vi "Set Metadata.vi"(9 "Metadata Disable":T2={"spectrometer"=enum."Disabled and Grayed Out", "sphere"=enum."Disabled and Grayed Out", "analyzer"=enum."Disabled and Grayed Out", "ampGainRange"=enum."Disabled and Grayed Out"}, 11 "Data Fields":T1={"operatorName"="", "project"="", "measurementType"="", "sphere"="", "spectrometer"="", "powerSource"="", "analyzer"="", "fixtureType"="", "lampType"="", "sourceType"="", "testOrientation"="", "model"="", "sample"="", "hours"=".csv", "Amp Gain Range"=""}) -> (3 "Metadata Out":string[][](array[string]))   [LabVIEW 2013]
uses:
  Metadata disable typedef.ctl
  Metadata typedef.ctl
panel:
  in  "Ready?":bool
  out "data string":string
  # "ambient temp (sphere)"
  # "ambient temp room"
  # "Fill out the follow data fields for each test. An error will be thrown if any data fields are missing.\nNew parameters for data fields can be added by right clicking, hitting \"properties\", then \"edit items\""
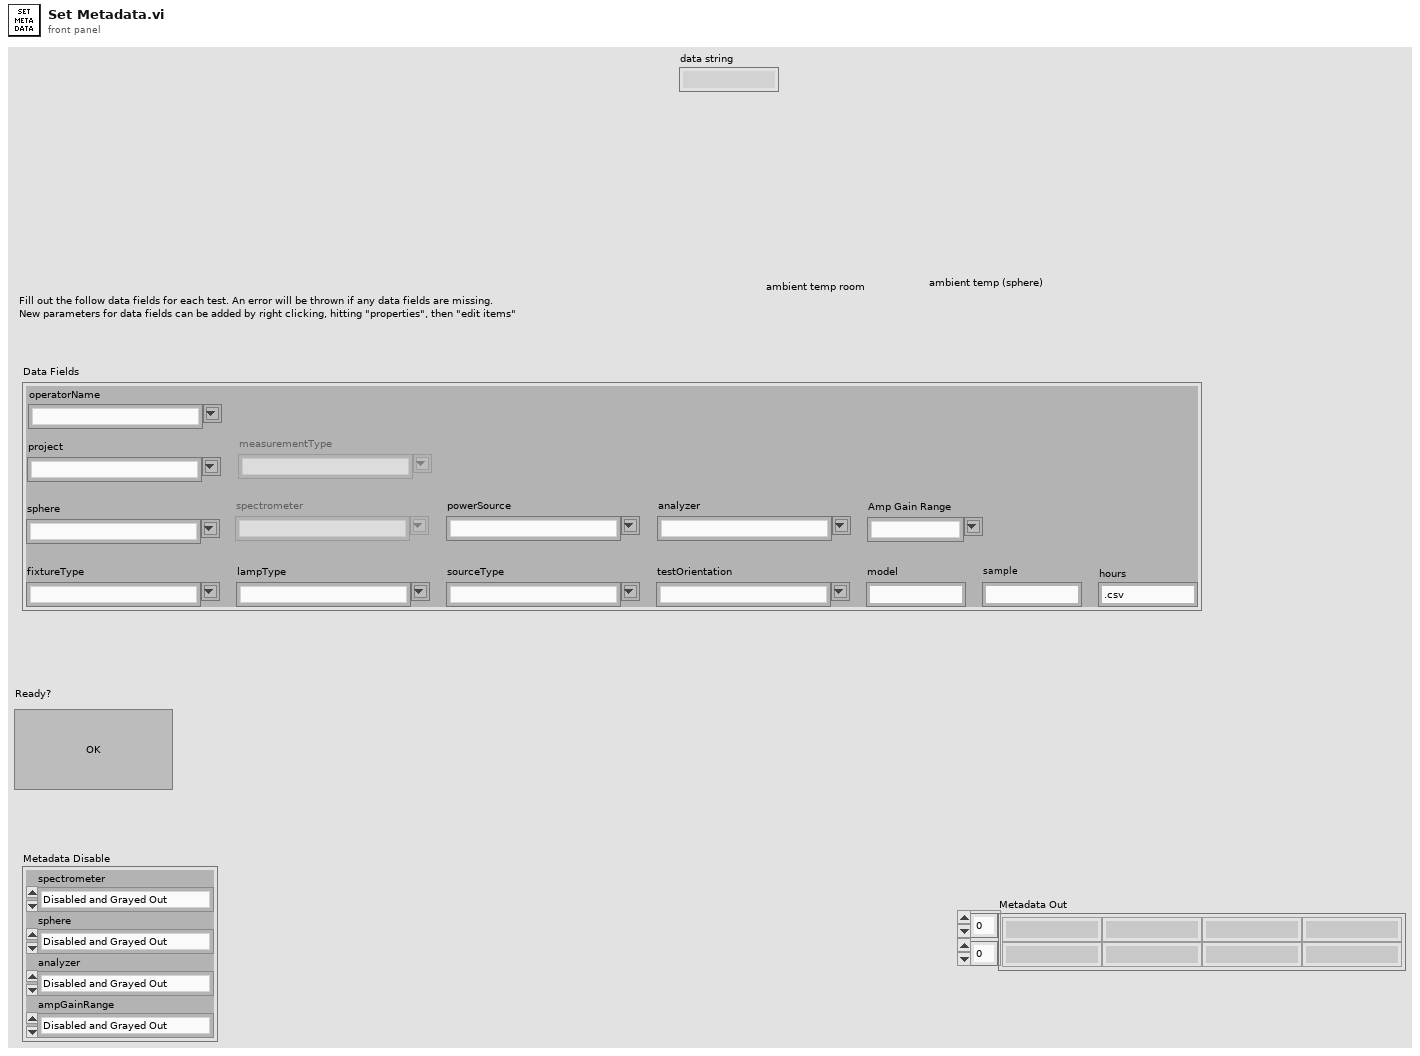
[diagram p1: front panel]
types:
  T1 = typedef "Metadata typedef.ctl" = cluster{"operatorName":string, "project":string, "measurementType":string, "sphere":string, "spectrometer":string, "powerSource":string, "analyzer":string, "fixtureType":string, "lampType":string, "sourceType":string, "testOrientation":string, "model":string, "sample":string, "hours":string, "Amp Gain Range":string}
  T2 = typedef "Metadata disable typedef.ctl" = cluster{"spectrometer":enum8{"Enabled", "Disabled", "Disabled and Grayed Out"}, "sphere":enum8{"Enabled", "Disabled", "Disabled and Grayed Out"}, "analyzer":enum8{"Enabled", "Disabled", "Disabled and Grayed Out"}, "ampGainRange":enum8{"Enabled", "Disabled", "Disabled and Grayed Out"}}
  T3 = enum8{"Enabled", "Disabled", "Disabled and Grayed Out"}
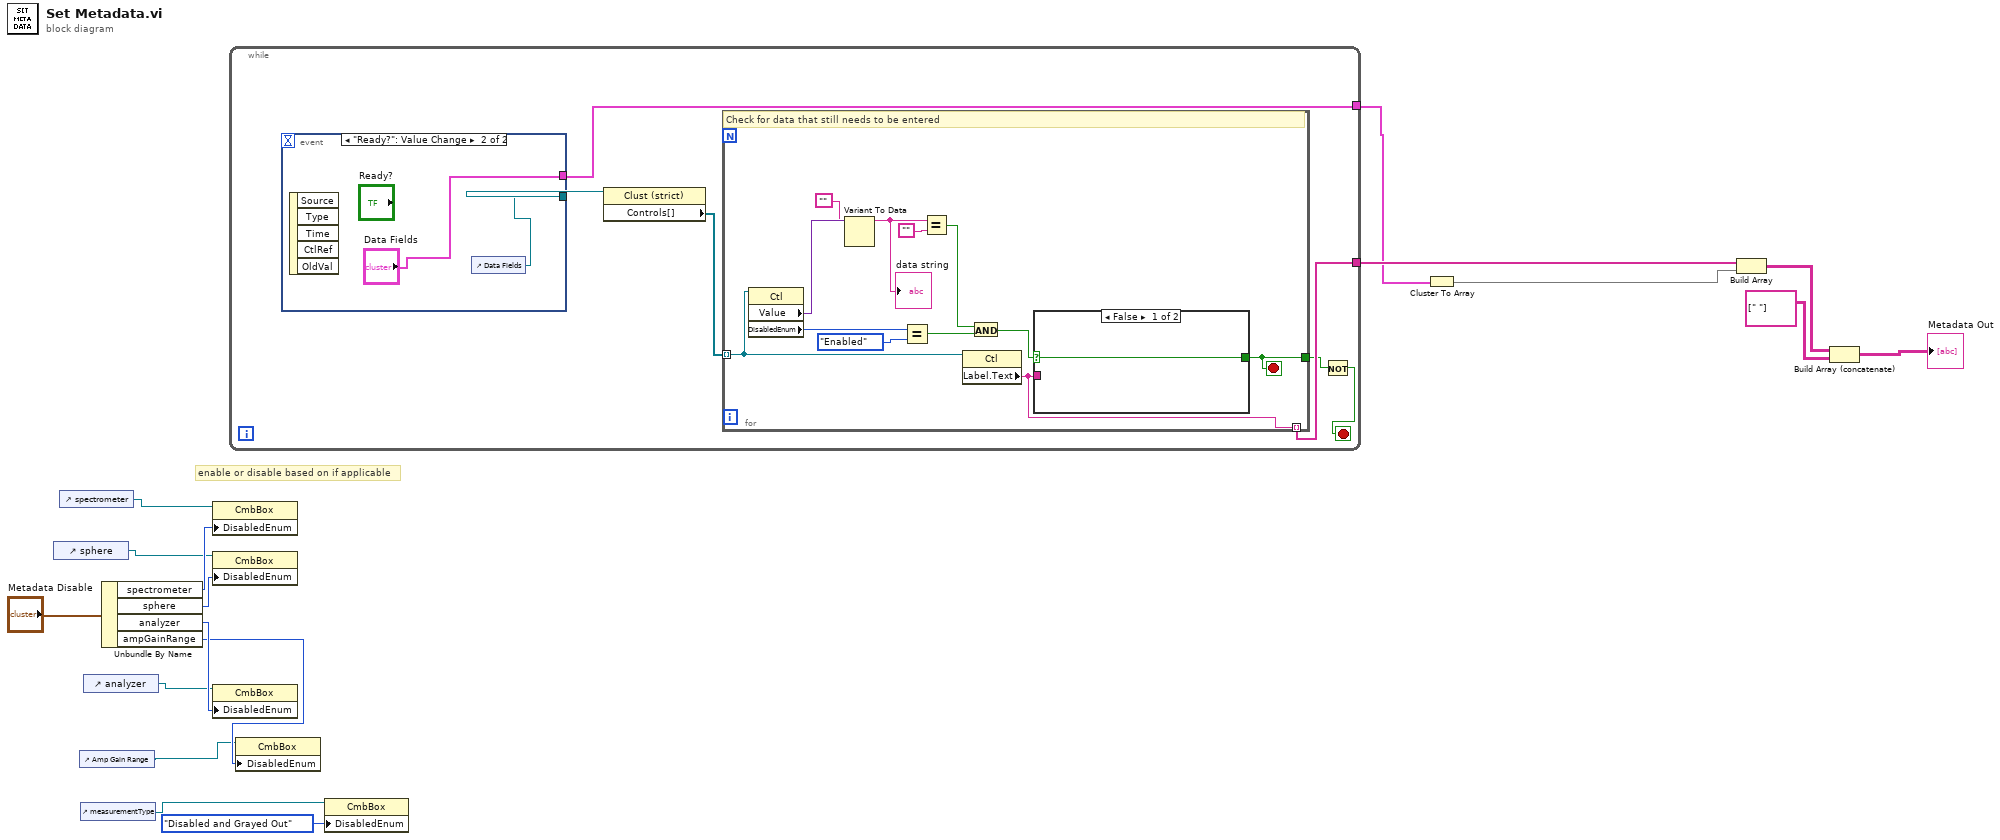
[diagram p0: block diagram]
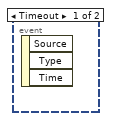
[diagram p2: hidden frame]
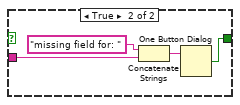
[diagram p3: hidden frame]
diagram:
  # "enable or disable based on if applicable"
  n1 = control-ref of="sphere"() -> (w2:refnum<vi>)
  n2 = control-ref of="spectrometer"() -> (w1:refnum<vi>)
  n3 = control-ref of="Amp Gain Range"() -> (w4:refnum<vi>)
  n4 = control-ref of="measurementType"() -> (w5:refnum<vi>)
  n5 = control-ref of="analyzer"() -> (w3:refnum<vi>)
  n6 = Unbundle By Name("Metadata Disable") -> ("spectrometer"=w15:T3, "sphere"=w14:T3, "analyzer"=w13:T3, "ampGainRange"=w7:T3)
  n7 = property class="CmbBox"(reference=w1, "DisabledEnum"=w15) -> ()  [unwired: 1 in, 2 out]
  n8 = property class="CmbBox"(reference=w2, "DisabledEnum"=w14) -> ()  [unwired: 1 in, 2 out]
  n9 = property class="CmbBox"(reference=w3, "DisabledEnum"=w13) -> ()  [unwired: 1 in, 2 out]
  n10 = while {
    tunnel: [w22] -> w17
    tunnel: [w20] -> w8
    stop <- w18 stop-if-true
    n11 = event shown="[1] \"Ready?\": Value Change" {
      selector: _ -> [_ _]
      dyn-events: _ -> [_ _]
      timeout: _ -> [_ _]
      tunnel: [_ w24] -> w21
      tunnel: [_ "Data Fields"] -> w20
      event Timeout {
        n12 = event-data() -> ()  [unwired: 1 in, 3 out]
      }
      event "Ready?": Value Change {
        n13 = event-data() -> ()  [unwired: 1 in, 5 out]
        n14 = control-ref of="Data Fields"() -> (w24:refnum<vi>)
      }
    }
    n15 = property class="Clust (strict)"(reference=w21) -> ("Controls[]"=w23:refnum<vi>[])  [unwired: 1 in, 2 out]
    n16 = for {
      tunnel: w23 -> [w34] mode=indexing
      tunnel: [w37] -> w19
      tunnel: [w31] -> w22 mode=indexing
      stop <- w37 stop-if-true
      # "Check for data that still needs to be entered"
      n17 = property class="Ctl"(reference=w34) -> ("Value"=w36:variant, "DisabledEnum"=w30:T3)  [unwired: 1 in, 2 out]
      n18 = Variant To Data(type="", Variant=w36) -> (data=w35:string)  [unwired: 1 in, 1 out]
      "data string" <- w35
      n19 = Equal?(x=w30, y=T3."Enabled" ("Disabled")) -> (x = y?=w26:bool)
      n20 = Equal?(x=w35, y="") -> (x = y?=w28:bool)
      n21 = property class="Ctl"(reference=w34) -> ("Label.Text"=w31:string)  [unwired: 1 in, 2 out]
      n22 = And(x=w28, y=w26) -> (x .and. y?=w27:bool)
      n23 = case shown="False" w27 {
        selector: w27 -> [w38 _]
        tunnel: w31 -> [_ w41]
        tunnel: [w38 w39] -> w37
        frame False {
        }
        frame True {
          n24 = Concatenate Strings("missing field for: ", w41) -> (w40:string)
          n25 = One Button Dialog(message=w40) -> (true=w39:bool)  [unwired: 1 in]
        }
      }
    }
    n26 = Not(x=w19) -> (.not. x?=w18:bool)
  }
  n27 = property class="CmbBox"(reference=w4, "DisabledEnum"=w7) -> ()  [unwired: 1 in, 2 out]
  n28 = property class="CmbBox"(reference=w5, "DisabledEnum"=T3."Disabled and Grayed Out" ("Disabled")) -> ()  [unwired: 1 in, 2 out]
  n29 = Cluster To Array(cluster=w8) -> (array=w10:string[])
  n30 = Build Array(w17, w10) -> (w12:string[][])
  n31 = Build Array (concatenate)(w12, string[][] [[" "]] ("array")) -> (→"Metadata Out":string[][])
